vi "Write Data to Std In.vi"(8 "error in":errorcluster, 10 "Data":u8[](array[numeric]), 11 "ASE Handle":refnum<class "ase.lvclass">) -> (0 "error out":errorcluster, 1 "State":T1, 3 "ASE Handle Duplicate":refnum<class "ase.lvclass">)   [LabVIEW 2024, in "serenial.io-ase.lvlib" / "ase.lvclass"]
doc: "<B>Write data (raw bytes) to the standard input.</B>\n\nThis VI generates the following errors:\n-5691000: Internal Library Error. Check Error Message for more details.\n1556: Invalid Handle Supplied"
uses:
  ase.lvclass
  Standard Input State.ctl
  ase.lvclass/ase.ctl
  Error Internal Library Implementation Error.vi
  <vilib>/Utility/error.llb/Error Cluster From Error Code.vi
  serenial.io-ase.32.dll
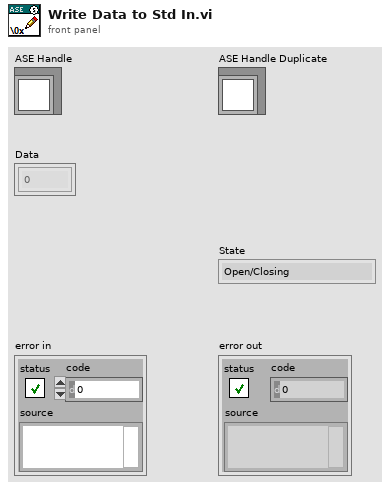
[diagram p1: front panel]
types:
  T1 = typedef "serenial.io-ase.lvlib/ase.lvclass/Standard Input State.ctl" = enum16{"Open/Closing", "Closed"}
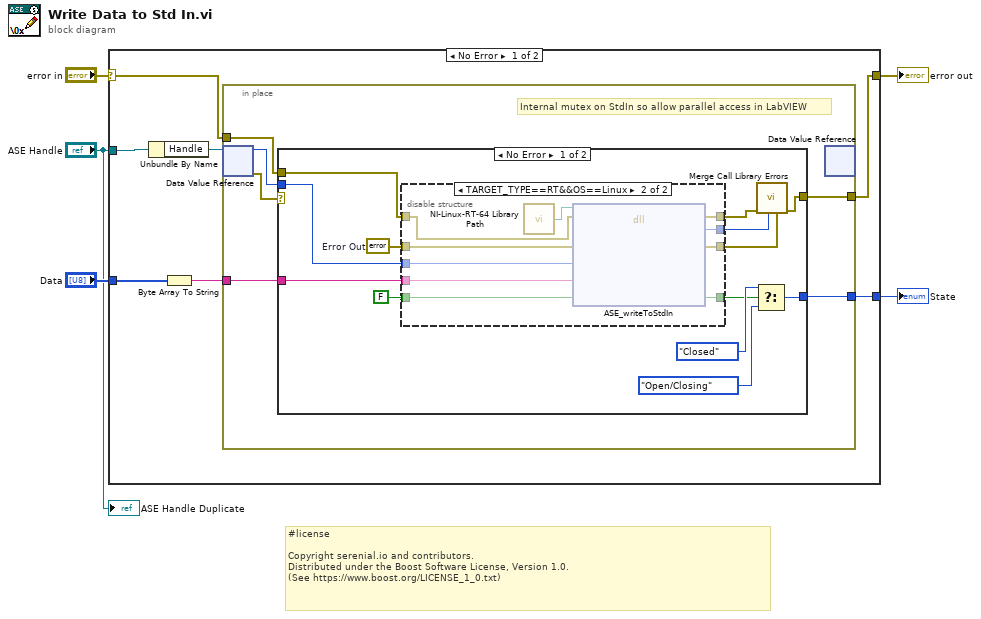
[diagram p0: block diagram]
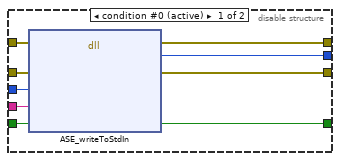
[diagram p2: hidden frame]
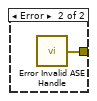
[diagram p3: hidden frame]
diagram:
  # "#license\n\nCopyright serenial.io and contributors.\nDistributed under the Boost Software License, Version 1.0.\n(See https://www.boost.org/LICENSE_1_0.txt)"
  n1 = case shown="No Error" "error in" {
    selector: "error in" -> [w12 w52]
    tunnel: [w9 w52] -> w4
    tunnel: "ASE Handle" -> [w7 _]
    tunnel: "Data" -> [w11 _]
    tunnel: [w8 _] -> w1
    frame No Error {
      n2 = Unbundle By Name(w7) -> ("Handle"=w6:refnum<data-value>)
      n3 = Byte Array To String(unsigned byte array=w11) -> (string=w10:string)
      n4 = in-place "In Place Element Structure" {
        in-place-border: w12 -> [w18]
        in-place-border: w10 -> [w16]
        in-place-border: [w15] -> w9
        in-place-border: [w14] -> w8
        # "Internal mutex on StdIn so allow parallel access in LabVIEW"
        n5 = in-place-dvr #1 ("Data Value Reference Read / Write Element")(w6) -> (w13:u64, w17:errorcluster)
        n6 = case shown="No Error" w17 {
          tunnel: w13 -> [w25 _]
          tunnel: w18 -> [w27 _]
          tunnel: w16 -> [w24 _]
          tunnel: [w31 w51] -> w15
          tunnel: [w28 _] -> w14
          frame No Error {
            w26 = errorcluster {"status"=FALSE, "code"=0, "source"=""}  # Error Out
            n7 = disable-structure "Conditional Disable Structure" shown="TARGET_TYPE==RT&&OS==Linux" {
              disable-tunnel: w27 -> [w40 w50]
              disable-tunnel: w26 -> [w39 w49]
              disable-tunnel: w25 -> [w38 w48]
              disable-tunnel: w24 -> [w37 w47]
              disable-tunnel: FALSE -> [w36 w46]
              disable-tunnel: [w35 w44] -> w22
              disable-tunnel: [w34 w43] -> w21
              disable-tunnel: [w33 w42] -> w20
              disable-tunnel: [w32 w45] -> w19
              frame condition #0 (active) {
                n8 = dll-call lib="C:/Users/marc/code/sift-streaming/labview/Sift/Dependencies/asynchronous-system-exec-v2.0.0/serenial.io-ase/ase/serenial.io-ase.*.*" fn="ASE_writeToStdIn"(error in=w40, "Error Out"=w39, "ASE interface"=w38, "Input"=w37, "Already Closed"=w36) -> (error out=w35:errorcluster, "Error Code"=w34:i32, "Error Out"=w33:errorcluster, "Already Closed"=w32:bool)  [unwired: 4 in, 1 out]
              }
              frame condition #1 {
                n9 = call "NI-Linux-RT-64 Library Path.vi"() -> ("Path"=w41:path)
                n10 = dll-call lib="?" fn="ASE_writeToStdIn"(path in=w41, error in=w50, "Error Out"=w49, "ASE interface"=w48, "Input"=w47, "Already Closed"=w46) -> (error out=w44:errorcluster, "Error Code"=w43:i32, "Error Out"=w42:errorcluster, "Already Closed"=w45:bool)  [unwired: 3 in, 1 out]
              }
            }
            n11 = Select(t=Standard_Input_State."Closed" ("State"), s=w19, f=Standard_Input_State."Open/Closing" ("State")) -> (s? t:f=w28:T1)
            n12 = call "Merge Call Library Errors.vi"("Library Call Returned Error"=w20, "Error Code"=w21, "error in"=w22) -> ("error IO"=w31:errorcluster)  [unwired: 8 in]
          }
          frame Error {
            n13 = call "Error Invalid ASE Handle.vi"() -> ("Invalid ASE Handle"=w51:errorcluster)
          }
        }
        n14 = in-place-dvr #1 ("Data Value Reference Read / Write Element")() -> ()  [unwired: 1 in, 2 out]
      }
    }
    frame Error {
    }
  }
  "error out" <- w4
  "State" <- w1
  "ASE Handle Duplicate" <- "ASE Handle"
